vi "Clear-object.vi"(8 "error in (no error)":errorcluster, 11 "SM1000-control":T1) -> (0 "error out":errorcluster, 3 "SM1000-control out":T1)   [LabVIEW 2013, in "MaterialCharacterization.lvlib" / "MC-SM1000.lvclass"]
uses:
  MC-SM1000.lvclass
  Object-reference.ctl
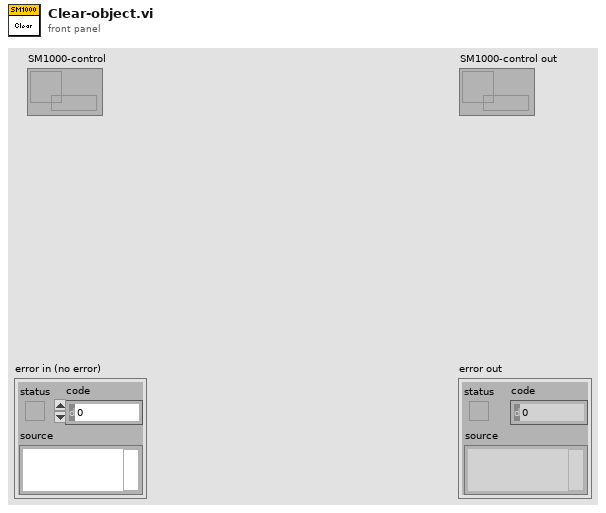
[diagram p1: front panel]
types:
  T1 = typedef "MaterialCharacterization.lvlib/MC-SM1000.lvclass/Object-reference.ctl" = refnum<data-value>
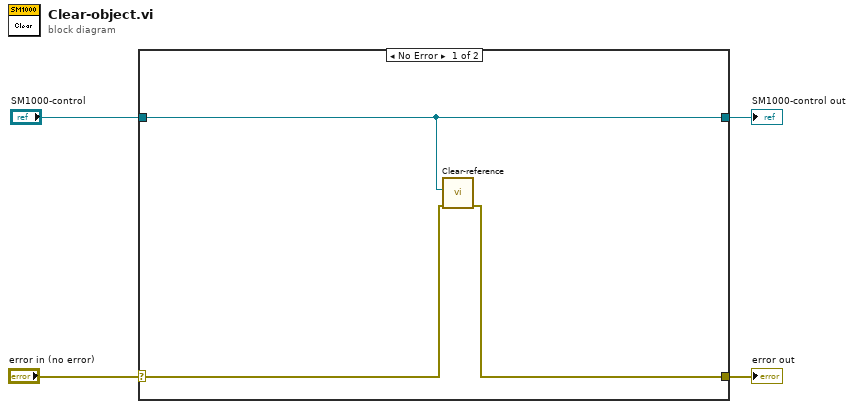
[diagram p0: block diagram]
diagram:
  n1 = case shown="No Error" "error in (no error)" {
    selector: "error in (no error)" -> [w6 w8]
    tunnel: [w5 w8] -> w3
    tunnel: [w7 _] -> w2
    tunnel: "SM1000-control" -> [w7 _]
    frame No Error {
      n2 = call "Clear-reference.vi"("error in (no error)"=w6, "Object reference"=w7) -> ("error out"=w5:errorcluster)  [unwired: 8 in, 1 out]
    }
    frame Error {
    }
  }
  "error out" <- w3
  "SM1000-control out" <- w2
